vi "XMLGetRows.vi"(11 "XML":string) -> (3 "Rows":string[](array[string]))   [LabVIEW 2014]
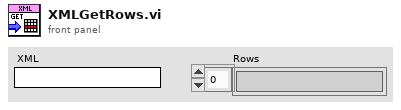
[diagram p1: front panel]
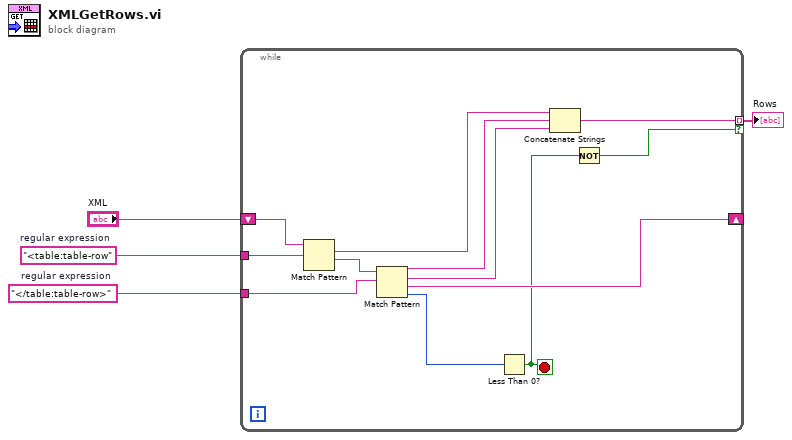
[diagram p0: block diagram]
diagram:
  w2 = "</table:table-row>"  # regular expression
  w1 = "<table:table-row"  # regular expression
  n1 = while {
    shift-right: [w11] -> _
    shift-left: "XML" -> [w16]
    tunnel: w1 -> [w15]
    tunnel: w2 -> [w13]
    tunnel: [w7] -> w3 mode=indexing if=w5
    stop <- w6 stop-if-true
    n2 = Match Pattern(string=w16, regular expression=w15) -> (match substring=w8:string, after substring=w14:string)  [unwired: 1 in, 2 out]
    n3 = Match Pattern(string=w14, regular expression=w13) -> (before substring=w9:string, match substring=w10:string, after substring=w11:string, offset past match=w12:i32)  [unwired: 1 in]
    n4 = Less Than 0?(x=w12) -> (x < 0?=w6:bool)
    n5 = Concatenate Strings(w8, w9, w10) -> (w7:string)
    n6 = Not(x=w6) -> (.not. x?=w5:bool)
  }
  "Rows" <- w3
